vi "Close.vi"(8 "error in (no error)":errorcluster, 11 "Serial in":refnum<class "Serial.lvclass">) -> (0 "error out":errorcluster, 3 "Serial out":refnum<class "Serial.lvclass">)   [LabVIEW 2024, in "Serial.lvclass"]
doc: "Serial.lvclass:Close.vi\n\nThis VI closes the Serial Port.\n\nInstrument Communication Module Version 1.0\nJuly, 2017 Original Code Consulting David Thomson\n www.originalcode.com"
uses:
  Serial.lvclass
  Serial.lvclass/Serial.ctl
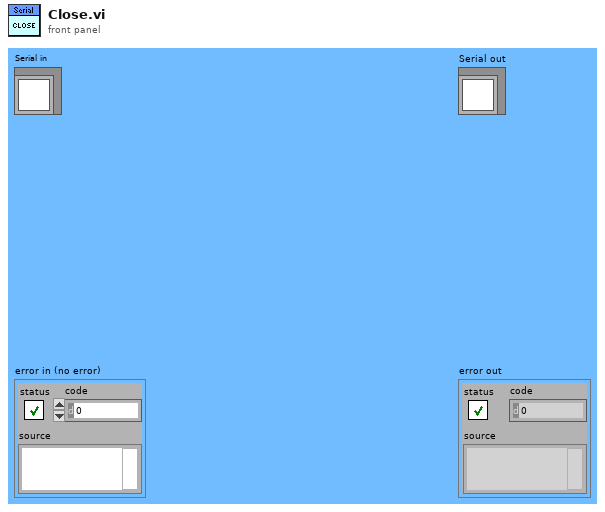
[diagram p1: front panel]
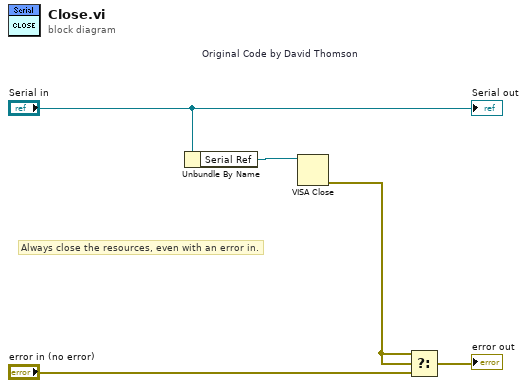
[diagram p0: block diagram]
diagram:
  # "Always close the resources, even with an error in."
  n1 = Unbundle By Name "Original Code by David Thomson"("Serial in") -> ("Serial Ref"=w4:refnum<visa-resource-name>)
  n2 = VISA Close(VISA resource name=w4) -> (error out=w2:errorcluster)  [unwired: 1 in]
  n3 = Select(t=w2, s=w2, f="error in (no error)") -> (s? t:f=→"error out":errorcluster)
  "Serial out" <- "Serial in"
